vi "Neg Binomial PF.vi"(9 "p":dbl=0.5, 10 "x":dbl=5.0, 11 "y":i32) -> (0 "error":i32, 3 "prob(y)":dbl=0.03125)   [LabVIEW 2010, in "NI_Gmath.lvlib"]
doc: "Computes the discrete probability function (PF), or the probability that the random variate X, where X describes the selected distribution type, takes on the value <B>n</B>. You must manually select the polymorphic instance to use."
uses:
  NI_Gmath.lvlib
panel:
  # "Negative Binomial PF"
  # "failures"
  # "successes"
  # "probability"
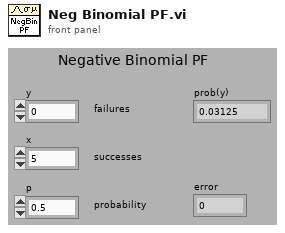
[diagram p1: front panel]
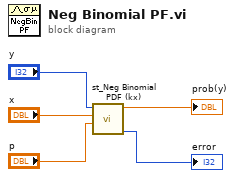
[diagram p0: block diagram]
diagram:
  n1 = call "st_Neg Binomial PDF (kx).vi"("p"="p", "x"="x", "ky"="y") -> ("error"=→"error":i32, "pdf(ky)"=→"prob(y)":dbl)  [unwired: 7 in]
